vi "MagX Logoff.vi"(8 "error in":errorcluster, 9 "Station":string="Cell_3", 10 "MagLab OSF tool server":string="magx.lanl.gov", 11 "Experiment ID":string="Cell_3") -> (0 "error out":errorcluster)   [LabVIEW 2021]
uses:
  <vilib>/httpClient/LabVIEWHTTPClient.lvlib
panel:
  out "body":string
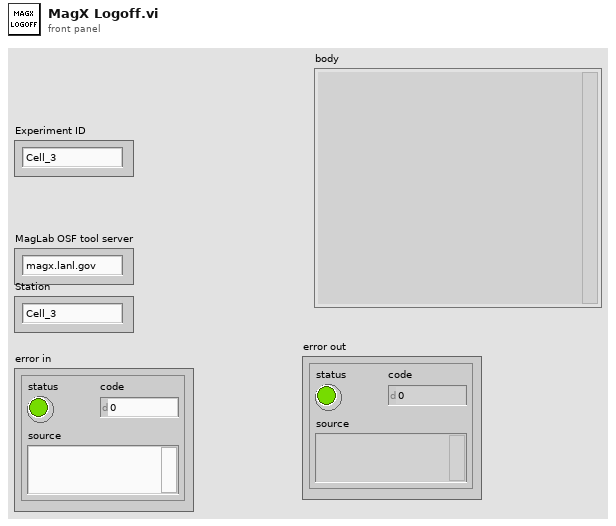
[diagram p1: front panel]
types:
  T1 = typedef "LabVIEWHTTPClient.lvlib/ClientHandle.ctl" = refnum<k1>
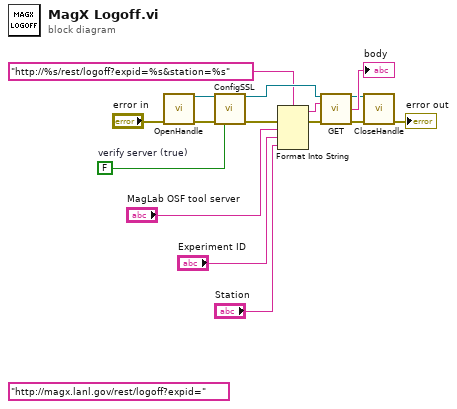
[diagram p0: block diagram]
diagram:
  (unwired) "http://magx.lanl.gov/rest/logoff?expid=" ("url")
  w11 = FALSE  # verify server (true)
  n1 = call <vilib>:"OpenHandle.vi"("error in (no error)"="error in") -> ("client handle out"=w14:T1, "error out"=w13:errorcluster)  [unwired: 13 in]
  n2 = call <vilib>:"ConfigSSL.vi"("client handle"=w14, "error in (no error)"=w13, "verify server (true)"=w11) -> ("client handle out"=w12:T1, "error out"=w2:errorcluster)  [unwired: 11 in]
  n3 = Format Into String(format string="http://%s/rest/logoff?expid=%s&station=%s" ("url"), error in=w2, "MagLab OSF tool server", "Experiment ID", "Station") -> (resulting string=w3:string, error out=w1:errorcluster)  [unwired: 1 in]
  n4 = call <vilib>:"GET.vi"("client handle"=w12, "url"=w3, "error in (no error)"=w1) -> ("client handle out"=w10:T1, "body"=→"body":string, "error out"=w9:errorcluster)  [unwired: 9 in, 1 out]
  n5 = call <vilib>:"CloseHandle.vi"("client handle"=w10, "error in (no error)"=w9) -> ("error out"=→"error out":errorcluster)  [unwired: 13 in]
